vi "test Parse DBL Array4.vi"(11 "Test Case In":refnum<class "Test Simple CSV Parser.lvclass">) -> (0 "error out":errorcluster, 3 "Test Case Out":refnum<class "Test Simple CSV Parser.lvclass">)   [LabVIEW 2024, in "Test Simple CSV Parser.lvclass"]
uses:
  Test Simple CSV Parser.lvclass
  Test Simple CSV Parser.lvclass/Test Simple CSV Parser.ctl
  CSV Parser/Simple CSV Parser/Simple CSV Parser.lvclass
  <vilib>/Astemes/LUnit/Test Case.lvclass
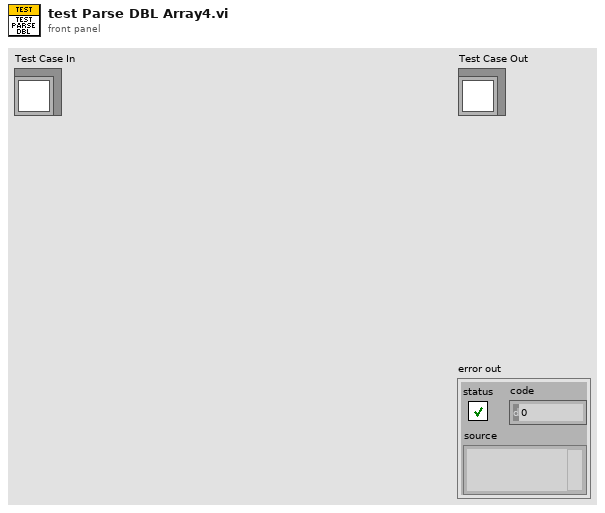
[diagram p1: front panel]
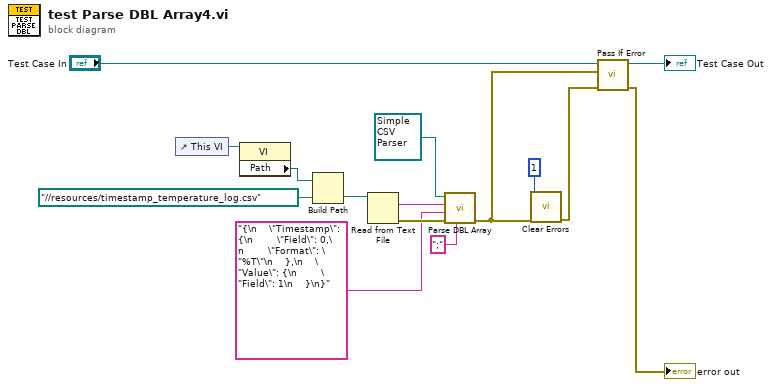
[diagram p0: block diagram]
diagram:
  n1 = control-ref of="This VI"() -> (w6:refnum<vi>)
  n2 = property class="VI"(reference=w6) -> ("Path"=w5:path)  [unwired: 1 in, 2 out]
  n3 = Build Path(base path=w5, name or relative path=path "../../resources/timestamp_temperature_log.csv" ("file (use dialog)")) -> (appended path=w8:path)
  n4 = Read from Text File(file (use dialog)=w8) -> (text=w3:string, error out=w4:errorcluster)  [unwired: 3 in, 2 out]
  n5 = call-dynamic "Parse DBL Array.vi"("Seperator"=";", "error in"=w4, "Input <JSON>"="{\n    \"Timestamp\": {\n        \"Field\": 0,\n        \"Format\": \"%T\"\n    },\n    \"Value\": {\n        \"Field\": 1\n    }\n}", "csv string"=w3, "Simple CSV Parser in"=refnum<class "Simple CSV Parser.lvclass"> refnum) -> ("error out"=w10:errorcluster)  [unwired: 4 in, 2 out]
  n6 = call <vilib>:"Clear Errors.vi"("error in (no error)"=w10, "specific error code to clear (0: all)"=1) -> ("error out"=w9:errorcluster)  [unwired: 4 in, 1 out]
  n7 = call <vilib>:"Pass If Error.vi"("error in (no error)"=w9, "Assert error"=w10, "LUnit Test Case In"="Test Case In") -> ("error out"=→"error out":errorcluster, "LUnit Test Case Out"=→"Test Case Out":refnum<class "Test Simple CSV Parser.lvclass">)  [unwired: 7 in]
